vi "ElemAreaGol.vi"(9 "AI Parameters":T1={"GotoKick"={"Dist do cone a frente"=0.0, "attacker farback"=1300.0, "Perto"=300.0, "min dist to kick"=140.0, "kick eps"=0.15, "Time to transition"=0.3}, "Attacker"={"CC chute"=0.7, "CC passe"=0.65, "Kick Force"=85.0, "ball-robot Kick"=300.0, "ball-robot Pass"=350.0, "drible\nAttk"=FALSE}, "Defender"={"D max"=1500.0, "Vel p/ robô av"=0.2, "Kick Force"=100.0, "D atk-def"=400.0, "D farback"=300.0, "drible\ndef"=FALSE, "drible\ngoalie"=FALSE}, "Timeout"={"Field/v in x"=6.0, "Dist Robots"=300, "Dist up in y"=300}, "Pose Striker"={"dist"=650.0, "Numeric"=-4.0, "dist 2"=650.0, "drible\nstriker"=TRUE}, "Dist Stop"=700.0, "D ball out"=200, "D central gap "=125.0, "T pass"=5.0, "Force ++"=5.0, "range kick"=60.0, "Chute alto"=TRUE, "Marcador novo"=TRUE, "drible"=FALSE, "D drible"=500.0, "Versão Striker"=enum."Auto", "Defesa"=enum."ManMark", "Marcador"=enum."Marcar o mais perigoso", "Receptor passe"=enum."Auto", "Área"=enum."Circular"} {"D drible" format="%#_13g"; "D central gap" format="%#_13g"; "Dist Stop" format="%#_13g"; "Pose Striker"."Numeric" format="%#_13g"; "Defender"."Kick Force" format="%#_13g"; "Defender"."Vel p/ robô av" format="%#_13g"; "Attacker"."ball-robot Kick" format="%#_13g"; "Attacker"."Kick Force" format="%#_13g"; "Attacker"."CC passe" format="%#_13g"; "Attacker"."CC chute" format="%#_13g"; "GotoKick"."min dist to kick" format="%#_13g"; "GotoKick"."Perto" format="%#_13g"; "GotoKick"."attacker farback" format="%#_13g"; "GotoKick"."Dist do cone a frente" format="%#_13g"}, 10 "IA State":T2={"our_robots"=[], "enemy_robots"=[], "balls"=[], "geometry"={"line_width"=0, "field_length"=0, "field_width"=0, "boundary_width"=0, "referee_width"=0, "goal_width"=0, "goal_depth"=0, "goal_wall_width"=0, "center_circle_radius"=0, "defense_radius"=0, "defense_stretch"=0, "free_kick_from_defense_dist"=0, "penalty_spot_from_field_line_dist"=0, "penalty_line_from_spot_dist"=0}, "IA Judge"={"stage"="", "command"="", "our_goalie_id"=0.0, "enemy_goalie_id"=0.0, "command enum"=enum."Halt", "Time"=enum."Azul"}, "Received Timestamp"=timestamp(0 s since 1904-01-01), "Events"={"Touch"=FALSE, "Ball out"=FALSE, "id touch"=0.0, "Ball out of \nVision"=FALSE, "Ball inside \nGoalie area"=FALSE, "Robot not responding"=FALSE, "Robots responding status"=[1.0, 1.0, 1.0, 1.0, 1.0, 1.0], "Enemy Ball \nPossession"=FALSE, "Pass State"=FALSE, "id end of pass"=0.0, "Kick"=FALSE, "Id ini Possession"=0.0, "Ball Possesion"=FALSE, "Id Possesion"=0.0, "Direct Kick"=FALSE, "2nd Strk Ativo"=FALSE}}, 11 "Elemento pos.":dbl[](array[numeric])) -> (2 "Elemento at goalkeeper area ?":bool)   [LabVIEW 2017]
uses:
  Core/AI Input.ctl
  Core/AI Robot.ctl
  Intel/Functions Enum.ctl
  Intel/AttackerStates.ctl
  Path Planning/RRT/PathDests.ctl
  Path Planning/RRT/PathDest.ctl
  Core/AI Ball.ctl
  Core/Field Size.ctl
  Core/AI Judge.ctl
  Intel/Command Enum.ctl
  Events/Events.ctl
  Intel/AI Parameters.ctl
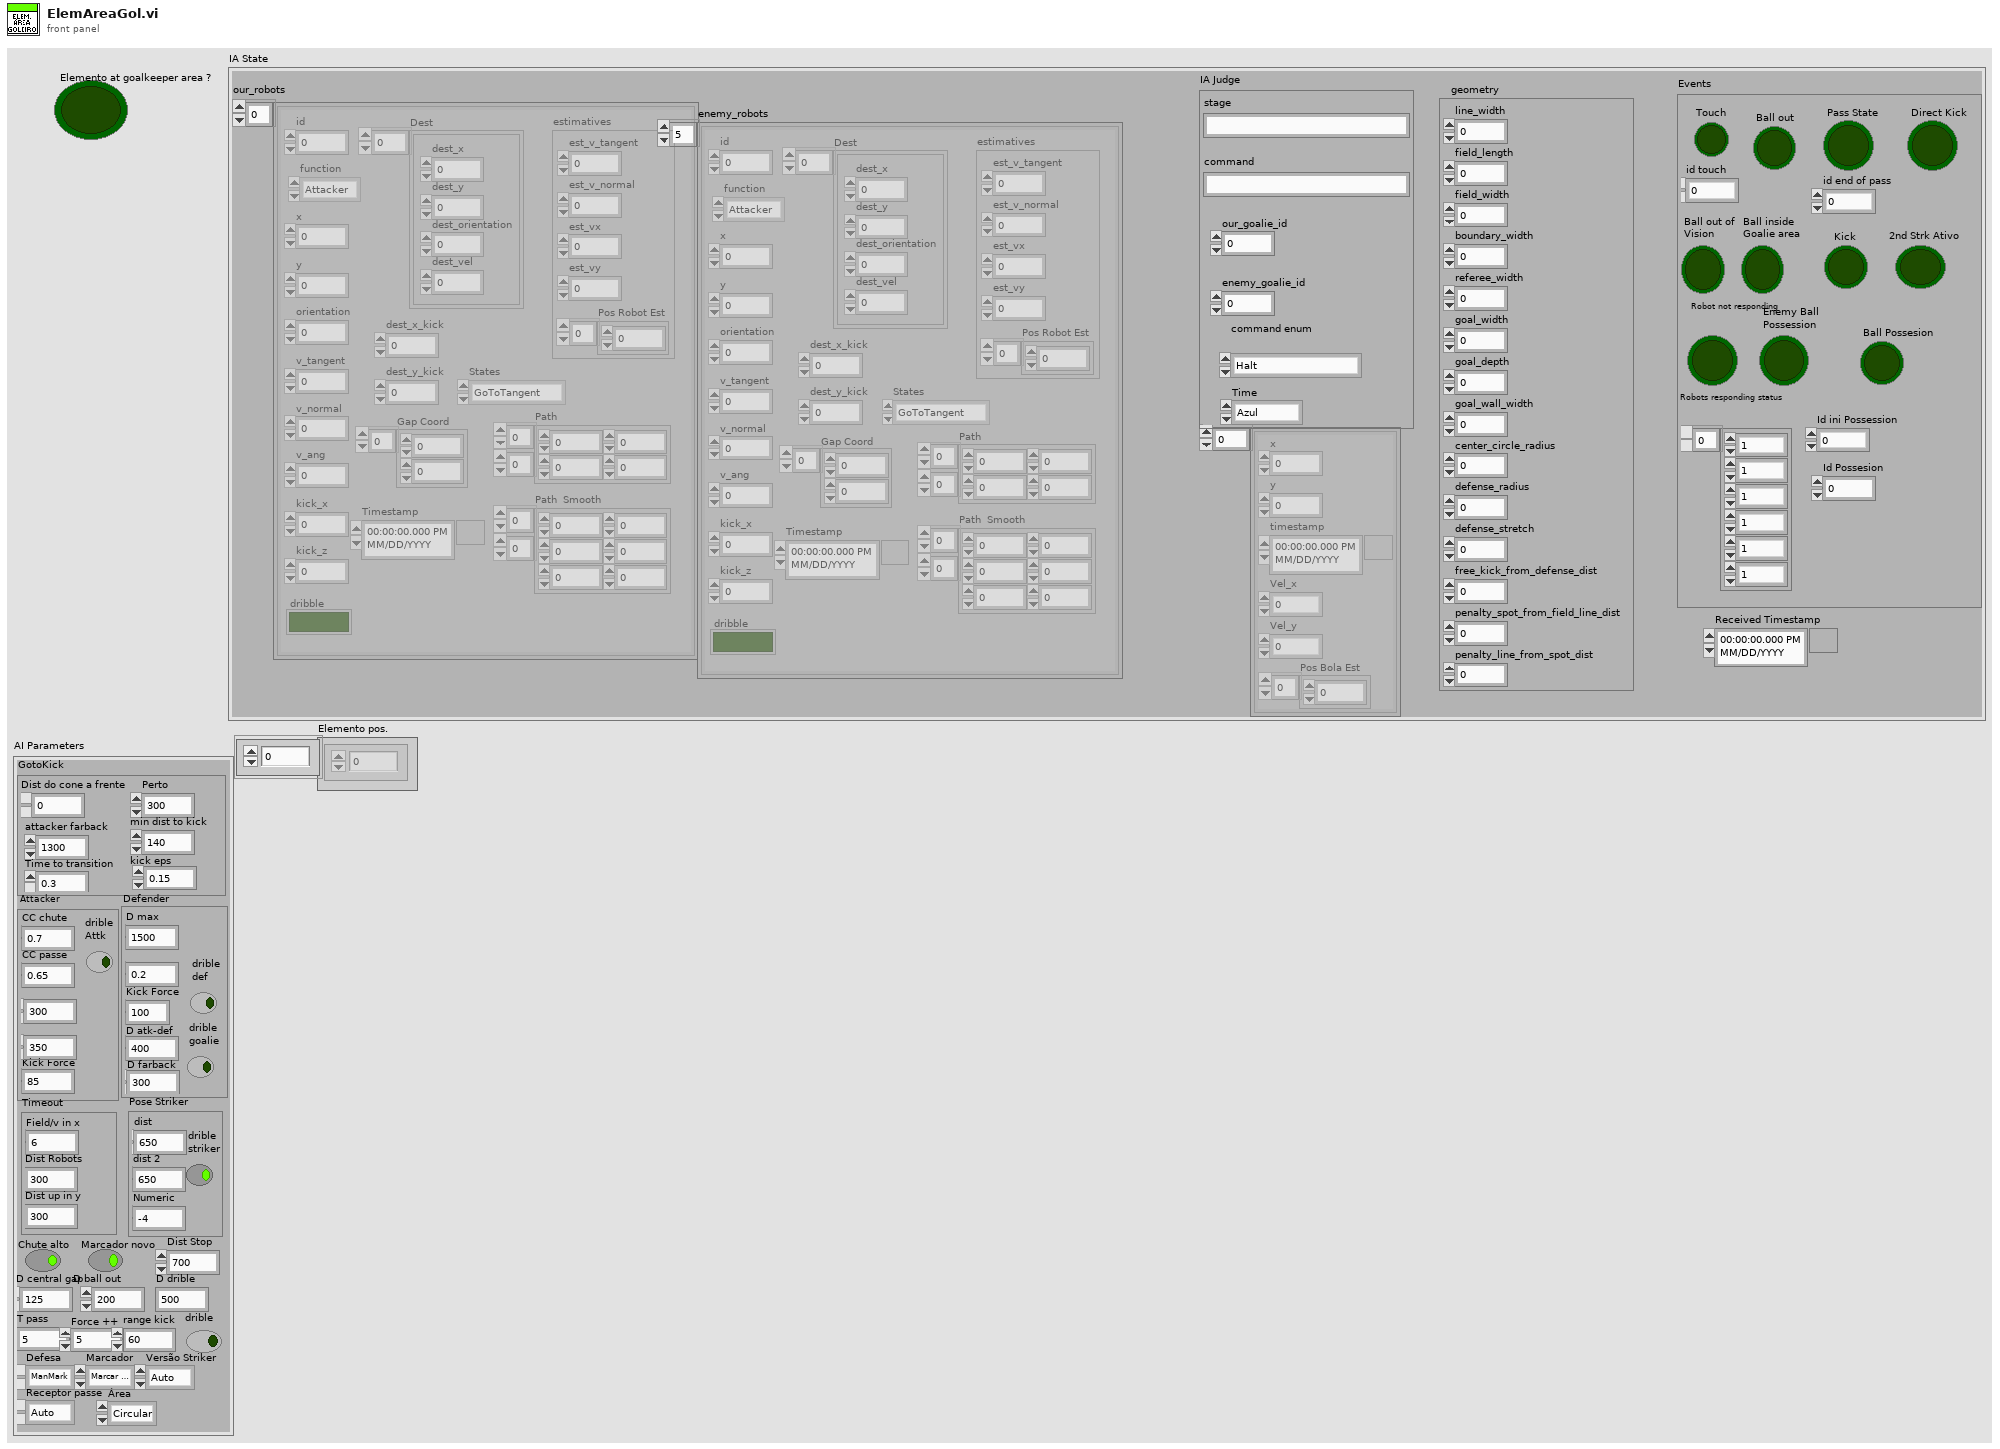
[diagram p1: front panel]
types:
  T1 = typedef "AI Parameters.ctl" = cluster{"GotoKick":cluster{"Dist do cone a frente":dbl, "attacker farback":dbl, "Perto":dbl, "min dist to kick":dbl, "kick eps":dbl, "Time to transition":dbl}, "Attacker":cluster{"CC chute":dbl, "CC passe":dbl, "Kick Force":dbl, "ball-robot Kick":dbl, "ball-robot Pass":dbl, "drible\nAttk":bool}, "Defender":cluster{"D max":dbl, "Vel p/ robô av":dbl, "Kick Force":dbl, "D atk-def":dbl, "D farback":dbl, "drible\ndef":bool, "drible\ngoalie":bool}, "Timeout":cluster{"Field/v in x":dbl, "Dist Robots":u32, "Dist up in y":u32}, "Pose Striker":cluster{"dist":dbl, "Numeric":dbl, "dist 2":dbl, "drible\nstriker":bool}, "Dist Stop":dbl, "D ball out":i32, "D central gap ":dbl, "T pass":dbl, "Force ++":dbl, "range kick":dbl, "Chute alto":bool, "Marcador novo":bool, "drible":bool, "D drible":dbl, "Versão Striker":enum16{"Auto", "3", "2", "1"}, "Defesa":enum16{"ManMark", "Barreira"}, "Marcador":enum16{"Marcar Segndo mais perigoso", "Marcar o mais perigoso"}, "Receptor passe":enum16{"Auto", "2nd Striker", "Striker"}, "Área":enum16{"Quadrada", "Circular"}}
  T2 = typedef "AI Input.ctl" = cluster{"our_robots":T3[], "enemy_robots":T3[], "balls":T8[], "geometry":T9, "IA Judge":T10, "Received Timestamp":timestamp, "Events":T12}
  T3 = typedef "AI Robot.ctl" = cluster{"id":u32, "function":T4, "x":dbl, "y":dbl, "orientation":dbl, "v_tangent":dbl, "v_normal":dbl, "v_ang":dbl, "kick_x":dbl, "kick_z":dbl, "dribble":bool, "Timestamp":timestamp, "estimatives":cluster{"est_v_tangent":dbl, "est_v_normal":dbl, "est_vx":dbl, "est_vy":dbl, "Pos Robot Est":dbl[]}, "dest_x_kick":dbl, "dest_y_kick":dbl, "Gap Coord":dbl[], "States":T5, "Path ":dbl[][], "Path  Smooth":dbl[][], "Dest":T6}
  T4 = typedef "Functions Enum.ctl" = enum16{"2nd Striker", "Attacker", "Goalie", "Defender", "Striker", "Goto 0", "Dummy", "Kicker", "ZigZag 0", "ZigZag 1", "ZigZag 2", "ZigZag 3", "ZigZag 4", "ZigZag 5", "ZigZag 6", "ZigZag 7", "ZigZag 8", ""}
  T5 = typedef "AttackerStates.ctl" = enum16{"Pass", "GoToTangent", "BallGetting", "GoToKick", ""}
  T6 = typedef "PathDests.ctl" = T7[]
  T7 = typedef "PathDest.ctl" = cluster{"dest_x":dbl, "dest_y":dbl, "dest_orientation":dbl, "dest_vel":dbl}
  T8 = typedef "AI Ball.ctl" = cluster{"x":dbl, "y":dbl, "timestamp":timestamp, "Vel_x":dbl, "Vel_y":dbl, "Pos Bola Est":dbl[]}
  T9 = typedef "Field Size.ctl" = cluster{"line_width":u32, "field_length":u32, "field_width":u32, "boundary_width":u32, "referee_width":u32, "goal_width":u32, "goal_depth":u32, "goal_wall_width":u32, "center_circle_radius":u32, "defense_radius":u32, "defense_stretch":u32, "free_kick_from_defense_dist":u32, "penalty_spot_from_field_line_dist":u32, "penalty_line_from_spot_dist":u32}
  T10 = typedef "AI Judge.ctl" = cluster{"stage":string, "command":string, "our_goalie_id":dbl, "enemy_goalie_id":dbl, "command enum":T11, "Time":enum16{"Azul", "Amarelo"}}
  T11 = typedef "Command Enum.ctl" = enum16{"Halt", "Stop", "Force Start", "PKA Normal Start", "Prepare Kickoff Ally", "PKE Normal Start", "Prepare Kickoff Enemy", "Prepare Penalty Ally", "PPA Normal Start", "Prepare Penalty Enemy", "PPE Normal Start", "Direct Free Enemy", "Direct Free Ally", "Indirect Free Enemy", "Indirect Free Ally", "Timeout Enemy", "Timeout Ally", "Goal Enemy", "Goal Ally", "Ball Placement Enemy", "Ball Placement Ally", "Normal Half Time", "Extra Time Break", "Extra Half Time", "None", "Post Game"}
  T12 = typedef "Events.ctl" = cluster{"Touch":bool, "Ball out":bool, "id touch":dbl, "Ball out of \nVision":bool, "Ball inside \nGoalie area":bool, "Robot not responding":bool, "Robots responding status":dbl[], "Enemy Ball \nPossession":bool, "Pass State":bool, "id end of pass":dbl, "Kick":bool, "Id ini Possession":dbl, "Ball Possesion":bool, "Id Possesion":dbl, "Direct Kick":bool, "2nd Strk Ativo":bool}
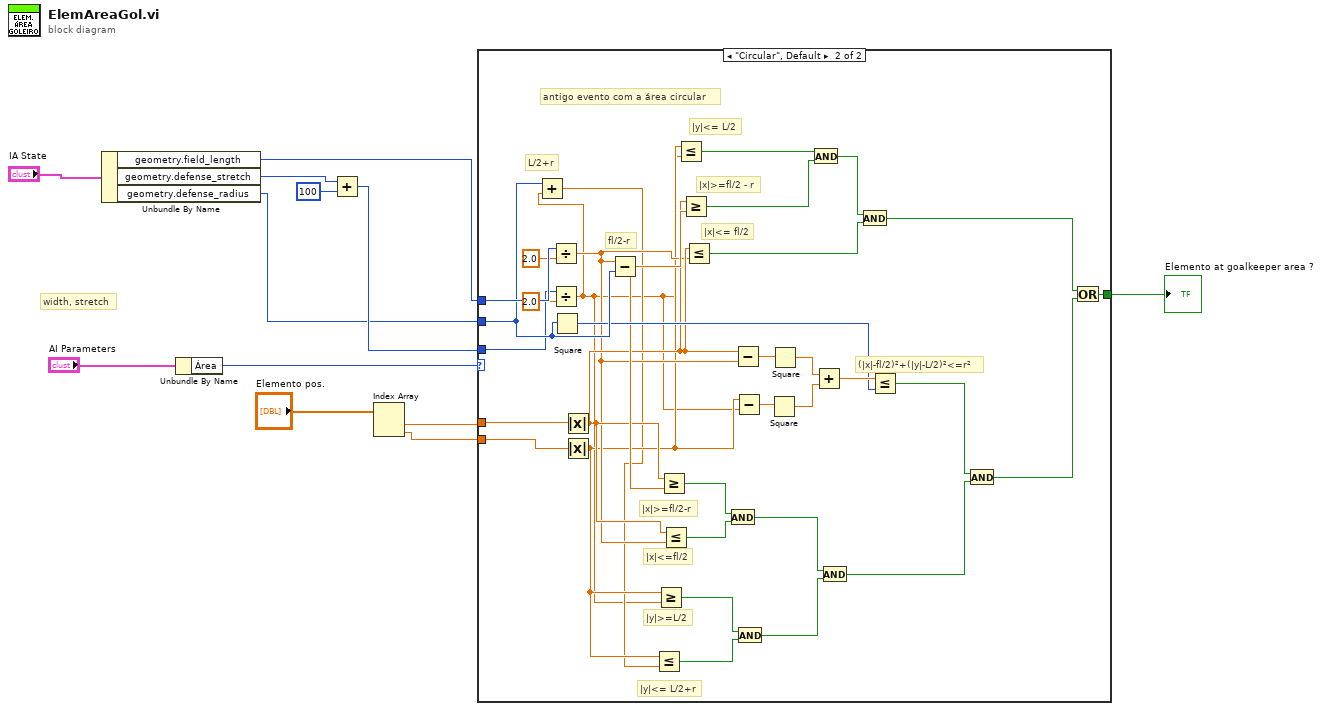
[diagram p0: block diagram]
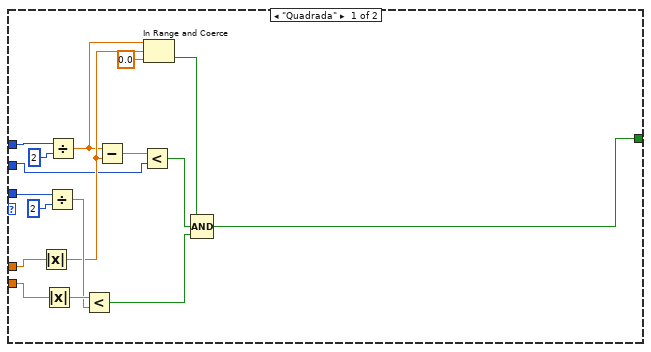
[diagram p2: hidden frame]
diagram:
  # "width, stretch"
  n1 = Unbundle By Name("IA State") -> ("geometry.field_length"=w4:u32, "geometry.defense_stretch"=w9:u32, "geometry.defense_radius"=w7:u32)
  n2 = Unbundle By Name("AI Parameters") -> ("Área"=w5:enum16{"Quadrada", "Circular"})
  n3 = Add(x=w9, y=u32 100) -> (x+y=w8:u32)
  n4 = Index Array(array="Elemento pos.") -> (element #1=w2:dbl, element #2=w3:dbl)  [unwired: 2 in]
  n5 = case shown="\"Circular\", Default" w5 {
    tunnel: w3 -> [w17 w63]
    tunnel: w2 -> [w18 w62]
    tunnel: w4 -> [w15 w61]
    tunnel: [w13 w60] -> w12
    tunnel: w7 -> [w14 w59]
    tunnel: w8 -> [w16 w58]
    frame "Quadrada" {
      n6 = Absolute Value(x=w18) -> (abs(x)=w22:dbl)
      n7 = Absolute Value(x=w17) -> (abs(x)=w28:dbl)
      n8 = Divide(x=w16, y=u32 2) -> (x/y=w25:dbl)
      n9 = Divide(x=w15, y=u32 2) -> (x/y=w20:dbl)
      n10 = Less?(x=w28, y=w25) -> (x < y?=w23:bool)
      n11 = Subtract(x=w20, y=w22) -> (x-y=w27:dbl)
      n12 = Less?(x=w27, y=w14) -> (x < y?=w24:bool)
      n13 = In Range and Coerce(upper limit=w20, x=w22, lower limit=0.0) -> (In Range?=w19:bool)  [unwired: 1 out]
      n14 = Compound Arithmetic op=AND(w19, w24, w23) -> (w13:bool)
    }
    frame "Circular", Default {
      # "antigo evento com a área circular"
      # "|y|<= L/2+r"
      # "L/2+r"
      # "|y|>=L/2"
      # "|x|<=fl/2"
      # "|x|>=fl/2-r"
      # "fl/2-r"
      # "(|x|-fl/2)²+(|y|-L/2)²<=r²"
      # "|x|<= fl/2"
      # "|x|>=fl/2 - r"
      # "|y|<= L/2"
      n15 = Divide(x=w61, y=2.0) -> (x/y=w41:dbl)
      n16 = Divide(x=w58, y=2.0) -> (x/y=w30:dbl)
      n17 = Add(x=w59, y=w30) -> (x+y=w39:dbl)
      n18 = Square(x=w59) -> (x^2=w46:u32)
      n19 = Absolute Value(x=w62) -> (abs(x)=w44:dbl)
      n20 = Absolute Value(x=w63) -> (abs(x)=w40:dbl)
      n21 = Subtract(x=w41, y=w59) -> (x-y=w45:dbl)
      n22 = Less Or Equal?(x=w40, y=w39) -> (x <= y?=w37:bool)
      n23 = Greater Or Equal?(x=w40, y=w30) -> (x >= y?=w38:bool)
      n24 = Greater Or Equal?(x=w44, y=w45) -> (x >= y?=w43:bool)
      n25 = Less Or Equal?(x=w44, y=w41) -> (x <= y?=w42:bool)
      n26 = Less Or Equal?(x=w40, y=w30) -> (x <= y?=w55:bool)
      n27 = Greater Or Equal?(x=w44, y=w45) -> (x >= y?=w54:bool)
      n28 = Less Or Equal?(x=w44, y=w41) -> (x <= y?=w52:bool)
      n29 = And(x=w43, y=w42) -> (x .and. y?=w36:bool)
      n30 = Subtract(x=w44, y=w41) -> (x-y=w51:dbl)
      n31 = Subtract(x=w40, y=w30) -> (x-y=w50:dbl)
      n32 = And(x=w38, y=w37) -> (x .and. y?=w35:bool)
      n33 = Square(x=w50) -> (x^2=w48:dbl)
      n34 = Square(x=w51) -> (x^2=w49:dbl)
      n35 = And(x=w55, y=w54) -> (x .and. y?=w53:bool)
      n36 = Add(x=w49, y=w48) -> (x+y=w47:dbl)
      n37 = And(x=w36, y=w35) -> (x .and. y?=w33:bool)
      n38 = And(x=w53, y=w52) -> (x .and. y?=w32:bool)
      n39 = Less Or Equal?(x=w47, y=w46) -> (x <= y?=w34:bool)
      n40 = And(x=w34, y=w33) -> (x .and. y?=w31:bool)
      n41 = Or(x=w32, y=w31) -> (x .or. y?=w60:bool)
    }
  }
  "Elemento at goalkeeper area ?" <- w12
